vi "Run_Core.vi"(0 "Message Popup in":refnum<class "Message Popup.lvclass">, 11 "error in (no error)":errorcluster) -> (4 "Message Popup out":refnum<class "Message Popup.lvclass">, 6 "Return":variant, 15 "error out":errorcluster)   [LabVIEW 2016, in "Message Popup.lvclass"]
uses:
  Message Popup.lvclass
  E:/Repository/LabVIEW Script Language/source code/LSL components/functions/functionsbase/functionbase.lvclass
  functionsbase/functionbase.lvclass/functionbase.ctl
  Message Popup.lvclass/Message Popup.ctl
  functionsbase/properties/Read Smart Syntax Representation.vi
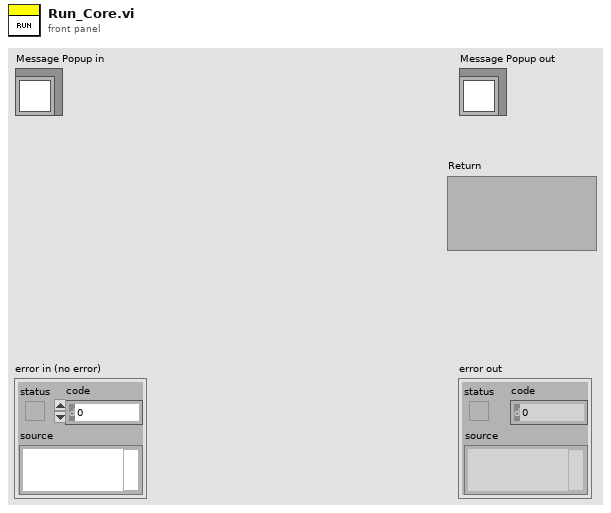
[diagram p1: front panel]
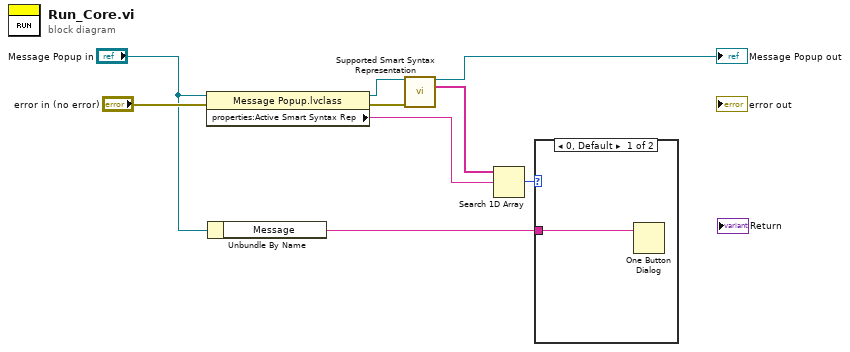
[diagram p0: block diagram]
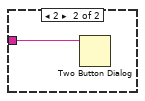
[diagram p2: hidden frame]
diagram:
  n1 = property class="Message Popup.lvclass"(reference="Message Popup in", error in="error in (no error)") -> (reference out=w5:refnum<class "Message Popup.lvclass">, error out=w8:errorcluster, "properties:Active Smart Syntax Rep"=w2:string)
  n2 = Unbundle By Name("Message Popup in") -> ("Message"=w1:string)
  n3 = call-dynamic "Supported Smart Syntax Representation.vi"("Message Popup in"=w5, "error in (no error)"=w8) -> ("Message Popup out"=→"Message Popup out":refnum<class "Message Popup.lvclass">, "Smart Syntax Representation List"=w7:string[])  [unwired: 11 in, 1 out]
  n4 = Search 1D Array(1D array=w7, element=w2) -> (index of element=w6:i32)  [unwired: 1 in]
  n5 = case shown="0, Default" w6 {
    tunnel: w1 -> [w10 w11]
    frame 0, Default {
      n6 = One Button Dialog(message=w10) -> ()  [unwired: 1 in, 1 out]
    }
    frame 2 {
      n7 = Two Button Dialog(message=w11) -> ()  [unwired: 2 in, 1 out]
    }
  }
